vi "get_offset.vi"(8 "error in (no error)":errorcluster, 11 "DL090503StimulatorScaffold.lvclass in":refnum<class "StimulatorDL090503Scaffold.lvclass">) -> (0 "error out":errorcluster, 2 "offset":dbl[unit], 3 "DL090503StimulatorScaffold.lvclass out":refnum<class "StimulatorDL090503Scaffold.lvclass">)   [LabVIEW 2010, in "StimulatorDL090503Scaffold.lvclass"]
uses:
  StimulatorDL090503Scaffold.lvclass
  StimulatorDL090503Scaffold.lvclass/StimulatorDL090503Scaffold.ctl
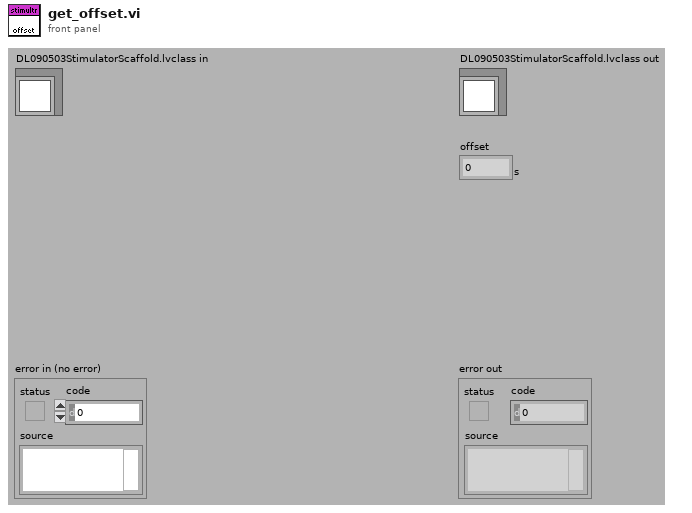
[diagram p1: front panel]
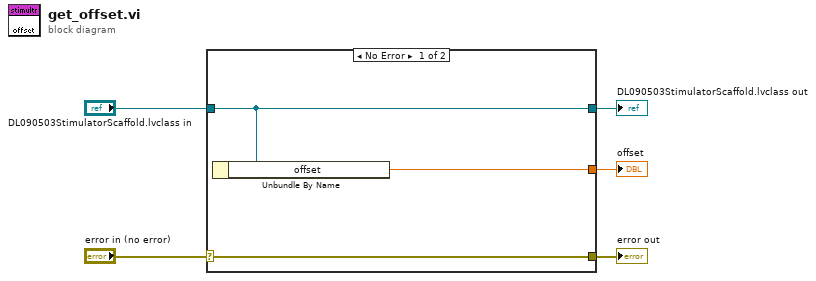
[diagram p0: block diagram]
diagram:
  n1 = case shown="No Error" "error in (no error)" {
    selector: "error in (no error)" -> [w8 w9]
    tunnel: [w8 w9] -> w4
    tunnel: [w7 w10] -> w2
    tunnel: "DL090503StimulatorScaffold.lvclass in" -> [w7 w10]
    tunnel: [w6 _] -> w1
    frame No Error {
      n2 = Unbundle By Name(w7) -> ("offset"=w6:dbl[unit])
    }
    frame Error {
    }
  }
  "error out" <- w4
  "DL090503StimulatorScaffold.lvclass out" <- w2
  "offset" <- w1
